vi "to_json.vi"(8 "error in":errorcluster, 11 "s3path in":refnum<class "s3path.lvclass">) -> (0 "error out":errorcluster, 2 "json":string, 3 "s3path out":refnum<class "s3path.lvclass">, 4 "Not Default":bool)   [LabVIEW 2020, in "nominal types.lvlib" / "timestampManifest.lvlib" / "s3path.lvclass"]
uses:
  s3path.lvclass
  s3path.lvclass/s3path.ctl
  07388e5c-2f37-468f-a409-5c4f42408061.vi
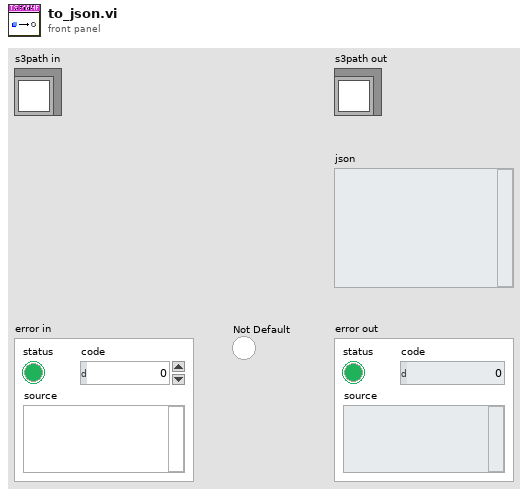
[diagram p1: front panel]
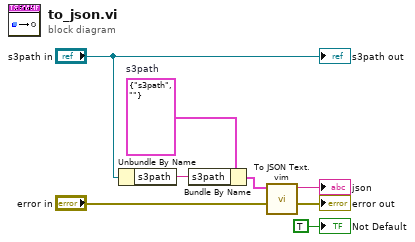
[diagram p0: block diagram]
diagram:
  w8 = cluster{"type":string, "s3path":string} {"type"="s3path", "s3path"=""}  # s3path
  n1 = Unbundle By Name("s3path in") -> ("s3path"=w7:string)
  n2 = Bundle By Name(cluster=w8, "s3path"=w7) -> (w6:cluster{"type":string, "s3path":string})
  n3 = call "To JSON Text.vim"("error in (no error)"="error in", "Anything"=w6) -> ("error out"=→"error out":errorcluster, "<JSON>"=→"json":string)  [unwired: 8 in]
  "s3path out" <- "s3path in"
  "Not Default" <- TRUE ("Not Default")
